vi "rad_UnForceSafeMode.vi"(8 "error in (no error)":errorcluster, 11 "Target in":refnum<k21>) -> (0 "error out":errorcluster, 3 "Target out":refnum<k21>)   [LabVIEW 2021]
uses:
  <vilib>/nisyscfg/Save Changes (Hardware).vi
  <vilib>/nisyscfg/Close (Hardware).vi
  <resource>/objmgr/nisysapi.rc
  <vilib>/nisyscfg/nisyscfg.lvlib
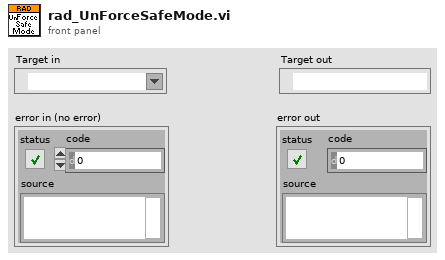
[diagram p1: front panel]
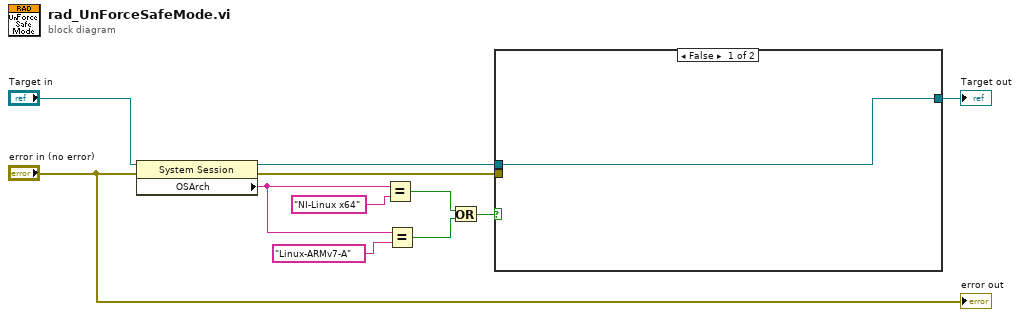
[diagram p0: block diagram]
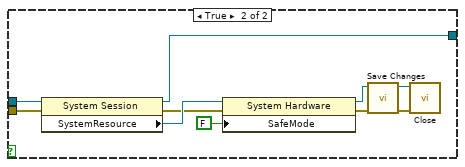
[diagram p2: hidden frame]
diagram:
  n1 = property class="System Session"(reference="Target in", error in="error in (no error)") -> (reference out=w3:refnum<k21>, error out=w4:errorcluster, "OSArch"=w10:string)
  n2 = Equal?(x=w10, y="NI-Linux x64") -> (x = y?=w7:bool)
  n3 = Equal?(x=w10, y="Linux-ARMv7-A") -> (x = y?=w6:bool)
  n4 = Or(x=w7, y=w6) -> (x .or. y?=w1:bool)
  n5 = case shown="False" w1 {
    tunnel: [w12 w22] -> w11
    tunnel: w4 -> [_ w14]
    tunnel: w3 -> [w12 w13]
    frame False {
    }
    frame True {
      n6 = property class="System Session"(reference=w13, error in=w14) -> (reference out=w22:refnum<k21>, error out=w20:errorcluster, "SystemResource"=w21:refnum<k20>)
      n7 = property class="System Hardware"(reference=w21, error in=w20, "SafeMode"=FALSE ("Startup Settings:User Directed Safe Mode")) -> (reference out=w17:refnum<k20>, error out=w18:errorcluster)
      n8 = call-poly <vilib>:"Save Changes.vi"("error in (no error)"=w18, "Resource in"=w17) -> ("error out"=w15:errorcluster, "Resource out"=w16:refnum<k20>)  [unwired: 6 in, 2 out]
      n9 = call-poly <vilib>:"Close.vi"("error in (no error)"=w15, "Resource in"=w16) -> ()  [unwired: 9 in, 1 out]
    }
  }
  "Target out" <- w11
  "error out" <- "error in (no error)"
